vi "NanonisFrame.vi"(0 "x":dbl, 1 "z":dbl) -> (8 "X Out":dbl, 10 "Z Out":dbl, 12 "Speed":dbl, 14 "FO X":dbl, 15 "FO Z":dbl, 16 "FW":dbl, 17 "FH":dbl, 19 "CVAL (nA)":dbl)   [LabVIEW 2019]
uses:
  <instrlib>/Nanonis Prog Interface V5/Nanonis Prog Interface.lvlib
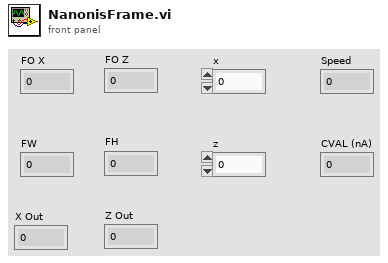
[diagram p1: front panel]
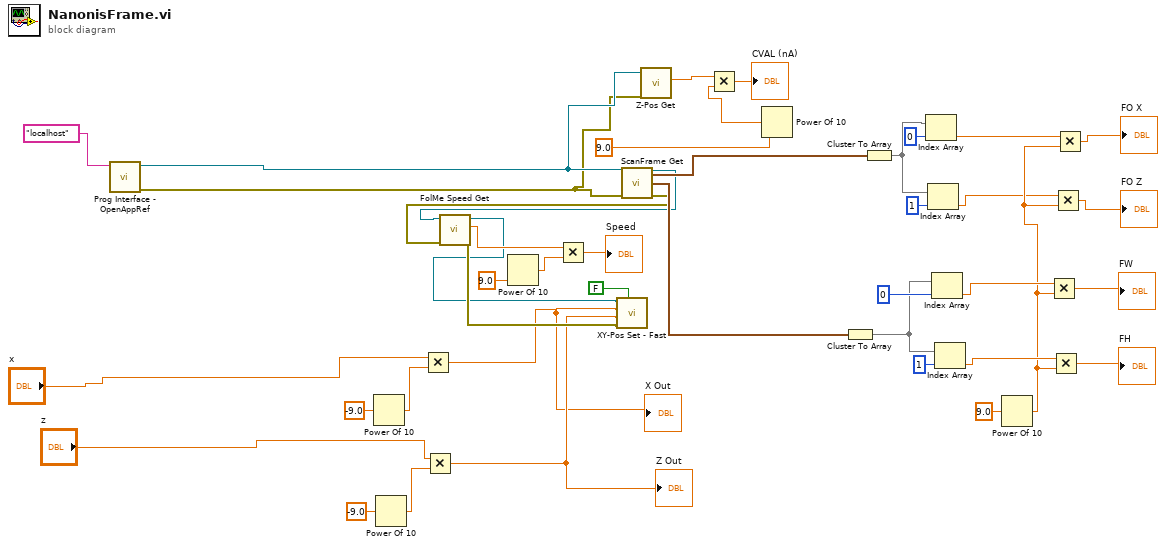
[diagram p0: block diagram]
diagram:
  n1 = call <instrlib>:"Prog Interface - OpenAppRef.vi"("Machine name (local machine IP)"="localhost") -> ("Error out"=w7:errorcluster, "Application reference"=w8:refnum<vi>)  [unwired: 5 in]
  n2 = Power Of 10(x=-9.0) -> (10^x=w22:dbl)
  n3 = Power Of 10(x=-9.0) -> (10^x=w20:dbl)
  n4 = Multiply(x="x", y=w22) -> (x*y=w3:dbl)
  "X Out" <- w3
  n5 = Multiply(x="z", y=w20) -> (x*y=w4:dbl)
  "Z Out" <- w4
  n6 = Power Of 10(x=9.0) -> (10^x=w25:dbl)
  n7 = call <instrlib>:"ScanFrame Get.vi"("Application ref in"=w8, "error in (no error)"=w7) -> ("Application ref out"=w27:refnum<vi>, "Center coordinates (m)"=w41:cluster{"Xc":sgl, "Yc":sgl}, "Size (m)"=w37:cluster{"Width":sgl, "Height":sgl}, "error out"=w18:errorcluster)  [unwired: 9 in, 1 out]
  n8 = call <instrlib>:"FolMe Speed Get.vi"("error in (no error)"=w18, "Application ref in"=w27) -> ("error out"=w5:errorcluster, "Speed (m/s)"=w24:sgl, "Application ref out"=w2:refnum<vi>)  [unwired: 4 in, 1 out]
  n9 = Multiply(x=w24, y=w25) -> (x*y=→"Speed":dbl)
  n10 = call <instrlib>:"XY-Pos Set - Fast.vi"("Wait end-of-motion (T=True)"=FALSE, "error in (no error)"=w5, "Y (m)"=w4, "X (m)"=w3, "Application ref in"=w2) -> ()  [unwired: 4 in, 2 out]
  n11 = call <instrlib>:"Z-Pos Get.vi"("error in (no error)"=w7, "Application ref in"=w8) -> ("Z position (m)"=w6:sgl)  [unwired: 7 in, 2 out]
  n12 = Power Of 10(x=9.0) -> (10^x=w10:dbl)
  n13 = Multiply(x=w6, y=w10) -> (x*y=→"CVAL (nA)":dbl)
  n14 = Cluster To Array(cluster=w37) -> (array=w34:sgl[])
  n15 = Cluster To Array(cluster=w41) -> (array=w40:sgl[])
  n16 = Index Array(array=w40, index=0) -> (element=w15:sgl)
  n17 = Index Array(array=w40, index=1) -> (element=w14:sgl)
  n18 = Index Array(array=w34, index=0) -> (element=w33:sgl)
  n19 = Index Array(array=w34, index=1) -> (element=w32:sgl)
  n20 = Power Of 10(x=9.0) -> (10^x=w30:dbl)
  n21 = Multiply(x=w33, y=w30) -> (x*y=→"FW":dbl)
  n22 = Multiply(x=w32, y=w30) -> (x*y=→"FH":dbl)
  n23 = Multiply(x=w14, y=w30) -> (x*y=→"FO Z":dbl)
  n24 = Multiply(x=w15, y=w30) -> (x*y=→"FO X":dbl)
